vi "Log Multiple Packets.vi"(8 "error in (no error)":errorcluster, 10 "Log Multiple Packets":T1[](array[typedef]), 11 "Log Sink in":refnum<class "Log Sink.lvclass">) -> (0 "error out":errorcluster, 3 "Log Sink out":refnum<class "Log Sink.lvclass">)   [LabVIEW 2018, in "MVA Framework.lvlib" / "Composed Log.lvlib" / "Log Sink.lvclass"]
uses:
  Log Sink.lvclass
  Types/Log Level.ctl
  Composed Log.lvlib
  Types/Log Packet.ctl
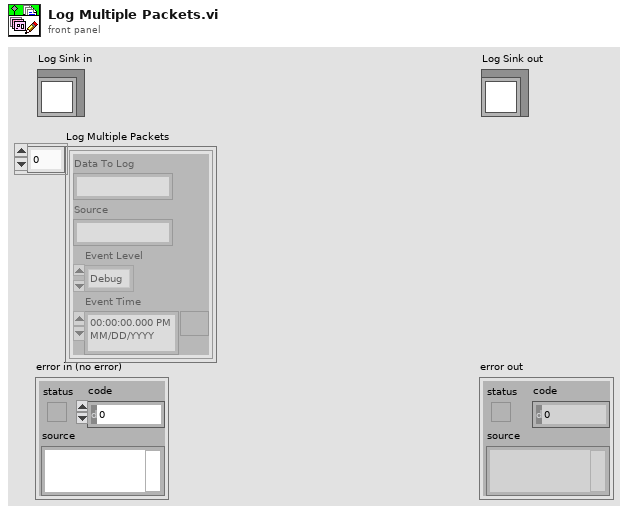
[diagram p1: front panel]
types:
  T1 = typedef "MVA Framework.lvlib/Composed Log.lvlib/Log Packet.ctl" = cluster{"Data To Log":string, "Source":string, "Event Level":T2, "Event Time":timestamp}
  T2 = typedef "MVA Framework.lvlib/Composed Log.lvlib/Log Level.ctl" = enum16{"Debug", "Info", "Warning", "Error", "Critical"}
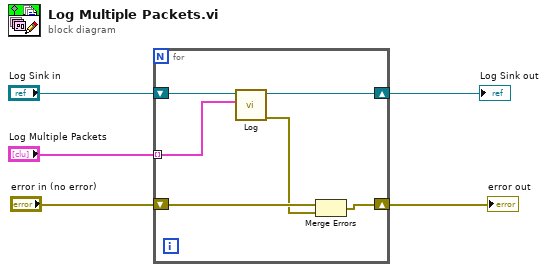
[diagram p0: block diagram]
diagram:
  n1 = for {
    shift-right: [w10] -> w4
    shift-left: "Log Sink in" -> [w11]
    tunnel: "Log Multiple Packets" -> [w9] mode=indexing
    shift-right: [w6] -> w1
    shift-left: "error in (no error)" -> [w8]
    n2 = call-dynamic "Log.vi"("Log Packet"=w9, "Log Sink in"=w11) -> ("error out"=w7:errorcluster, "Log Sink out"=w10:refnum<class "Log Sink.lvclass">)  [unwired: 8 in]
    n3 = Merge Errors(w8, w7) -> (w6:errorcluster)
  }
  "error out" <- w1
  "Log Sink out" <- w4
